vi "Update Remove Channel.vi"(5 "Display State In":T4={"Current Channels Info"=[], "Help Prefix"="", "Max Display Size"=8, "Max Size"=8, "Show Buttons"=TRUE, "Data Valid"=refnum, "Show Range"=FALSE, "Range Items"=[], "Range Index"=[]} caption="State", 7 "Channels In":T1, 8 "error in (no error)":errorcluster, 11 "Remove Channel Reference":refnum<vi>) -> (0 "error out":errorcluster)   [LabVIEW 2021, in "myRIO Channel List.xctl"]
uses:
  <vilib>/myRIO/Common/Express VI Framework/xctls/myRIO Channel List/myRIO Channel List.xctl
  <vilib>/myRIO/Common/Express VI Framework/xctls/myRIO Channel List/State.ctl
  <vilib>/myRIO/Common/Profile Manager Framework/typedefs/Channel Info.ctl
  <vilib>/myRIO/Common/Express VI Framework/typedefs/Data Validate Ref.ctl
  <vilib>/myRIO/Common/Express VI Framework/xctls/myRIO Channel List/Data.ctl
  <vilib>/myRIO/Common/Express VI Framework/xctls/myRIO Channel List/typedefs/Channel Data.ctl
  <vilib>/myRIO/Common/Express VI Framework/xctls/myRIO Channel List/typedefs/Remove Channel.ctl
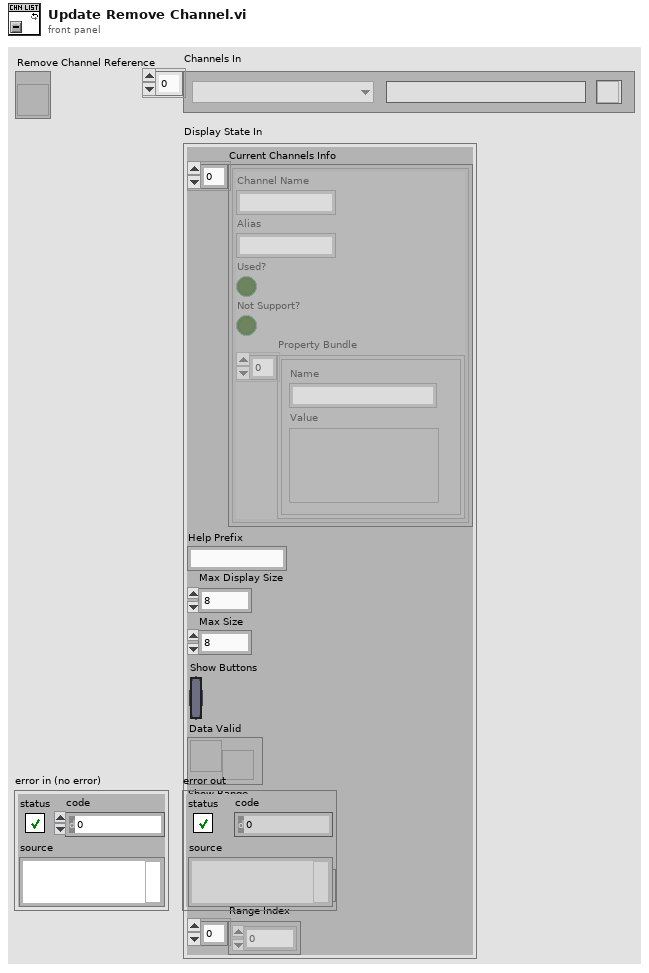
[diagram p1: front panel]
types:
  T1 = typedef "myRIO Channel List.xctl/Data.ctl" = T2[]
  T2 = typedef "myRIO Channel List.xctl/Channel Data.ctl" = cluster{"Channel Name":u16, "Channel Alias":string, "Remove Channel":T3, "Index":i32}
  T3 = typedef "myRIO Channel List.xctl/Remove Channel.ctl" = bool
  T4 = typedef "myRIO Channel List.xctl/State.ctl" = cluster{"Current Channels Info":T5[], "Help Prefix":string, "Max Display Size":i32, "Max Size":i32, "Show Buttons":bool, "Data Valid":T6, "Show Range":bool, "Range Items":string[], "Range Index":i32[]}
  T5 = typedef "Channel Info.ctl" = cluster{"Channel Name":string, "Alias":string, "Used?":bool, "Not Support?":bool, "Property Bundle":cluster{"Name":string, "Value":variant}[]}
  T6 = typedef "Data Validate Ref.ctl" = refnum<user-event>
  T7 = enum8{"Enabled", "Disabled", "Disabled and Grayed Out"}
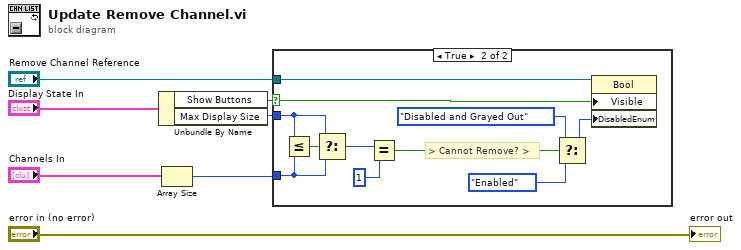
[diagram p0: block diagram]
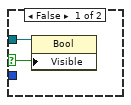
[diagram p2: hidden frame]
diagram:
  n1 = Unbundle By Name("Display State In") -> ("Show Buttons"=w4:bool, "Max Display Size"=w6:i32)
  n2 = Array Size(array="Channels In") -> (size(s)=w5:i32)
  n3 = case shown="True" w4 {
    selector: w4 -> [w8 w18]
    tunnel: w6 -> [_ w17]
    tunnel: w5 -> [_ w16]
    tunnel: "Remove Channel Reference" -> [w9 w20]
    frame False {
      n4 = property class="Bool"(reference=w9, "Visible"=w8) -> ()  [unwired: 1 in, 2 out]
    }
    frame True {
      # "> Cannot Remove? >"
      n5 = Less Or Equal?(x=w17, y=w16) -> (x <= y?=w19:bool)
      n6 = Select(t=w17, s=w19, f=w16) -> (s? t:f=w15:i32)
      n7 = Equal?(x=w15, y=1) -> (x = y?=w14:bool)
      n8 = Select(t=T7."Disabled and Grayed Out" ("Disabled"), s=w14, f=T7."Enabled" ("Disabled")) -> (s? t:f=w11:T7)
      n9 = property class="Bool"(reference=w20, "Visible"=w18, "DisabledEnum"=w11) -> ()  [unwired: 1 in, 2 out]
    }
  }
  "error out" <- "error in (no error)"
